vi "Experiment 12.vi"() -> ()   [LabVIEW 2026]
doc: "Experiment 12"
uses:
  <vilib>/AdvancedString/1D String Array to Delimited String (string).vi
  <vilib>/Analysis/baseanly.llb/Mean (DBL).vi
  <vilib>/Analysis/NI_AALBase.lvlib
panel:
  out "No. Of Iterations As Block Of Text (easy to copy into Excel)":string
  out "No. Of Iterations Executed - Loop 10":i32
  out "Output - Loop 10":dbl[](array[numeric]) format="%.3f"
  out "No. Of Iterations Executed - Loop 9":i32
  out "Output - Loop 9":dbl[](array[numeric]) format="%.3f"
  out "No. Of Iterations Executed - Loop 8":i32
  out "Output - Loop 8":dbl[](array[numeric]) format="%.3f"
  out "No. Of Iterations Executed - Loop 7":i32
  out "Output - Loop 7":dbl[](array[numeric]) format="%.3f"
  out "No. Of Iterations Executed - Loop 6":i32
  out "Output - Loop 6":dbl[](array[numeric]) format="%.3f"
  out "No. Of Iterations Executed - Loop 5":i32
  out "Output - Loop 5":dbl[](array[numeric]) format="%.3f"
  out "No. Of Iterations Executed - Loop 4":i32
  out "Output - Loop 4":dbl[](array[numeric]) format="%.3f"
  out "No. Of Iterations Executed - Loop 3":i32
  out "Output - Loop 3":dbl[](array[numeric]) format="%.3f"
  out "Avg. No. Of Iterations Executed - All Loops":dbl format="%.1f"
  out "No. Of Iterations Executed - Loop 2":i32
  out "Output - Loop 2":dbl[](array[numeric]) format="%.3f"
  out "No. Of Iterations Executed - Loop 1":i32
  out "Output - Loop 1":dbl[](array[numeric]) format="%.3f"
  out "Stop VI?":bool
  # "Experiment 12"
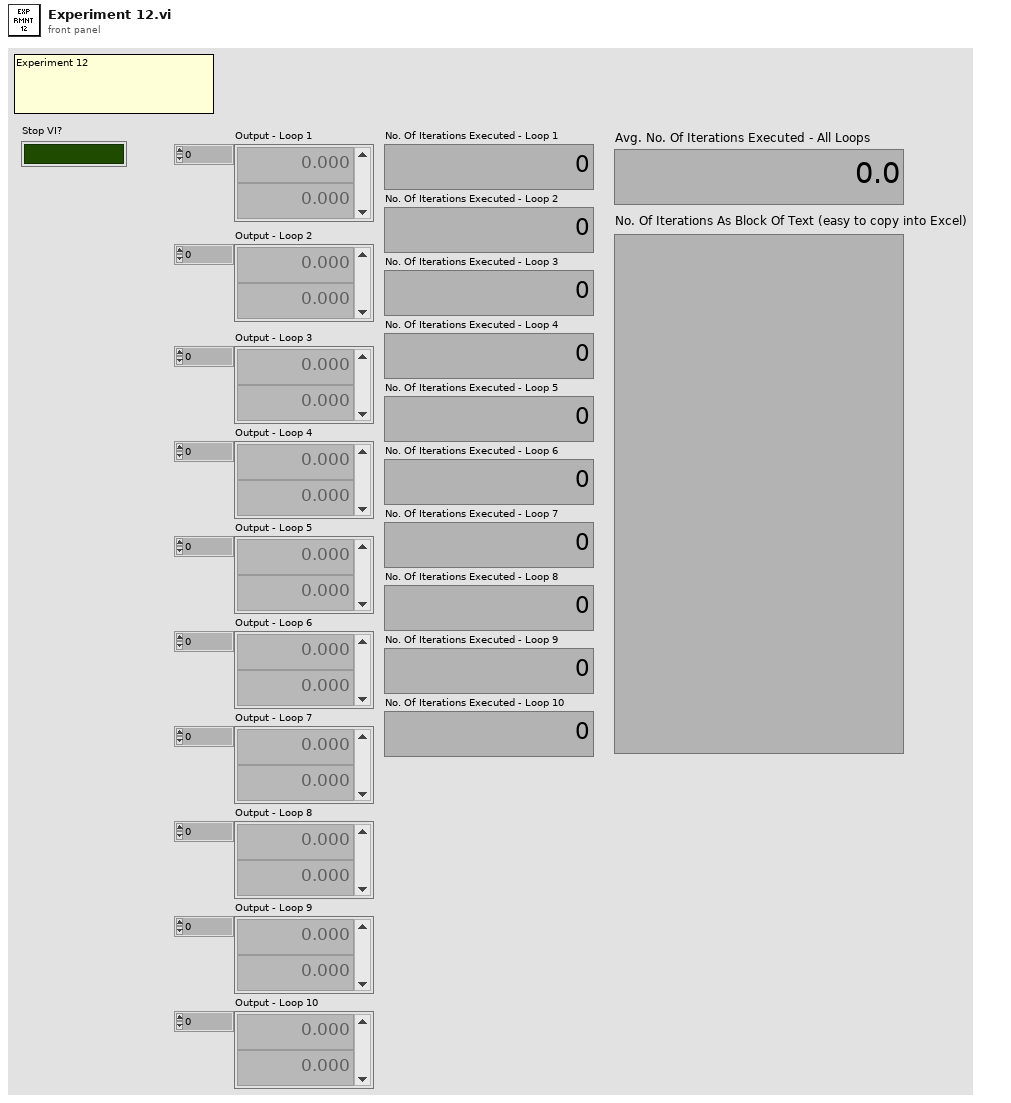
[diagram p1: front panel]
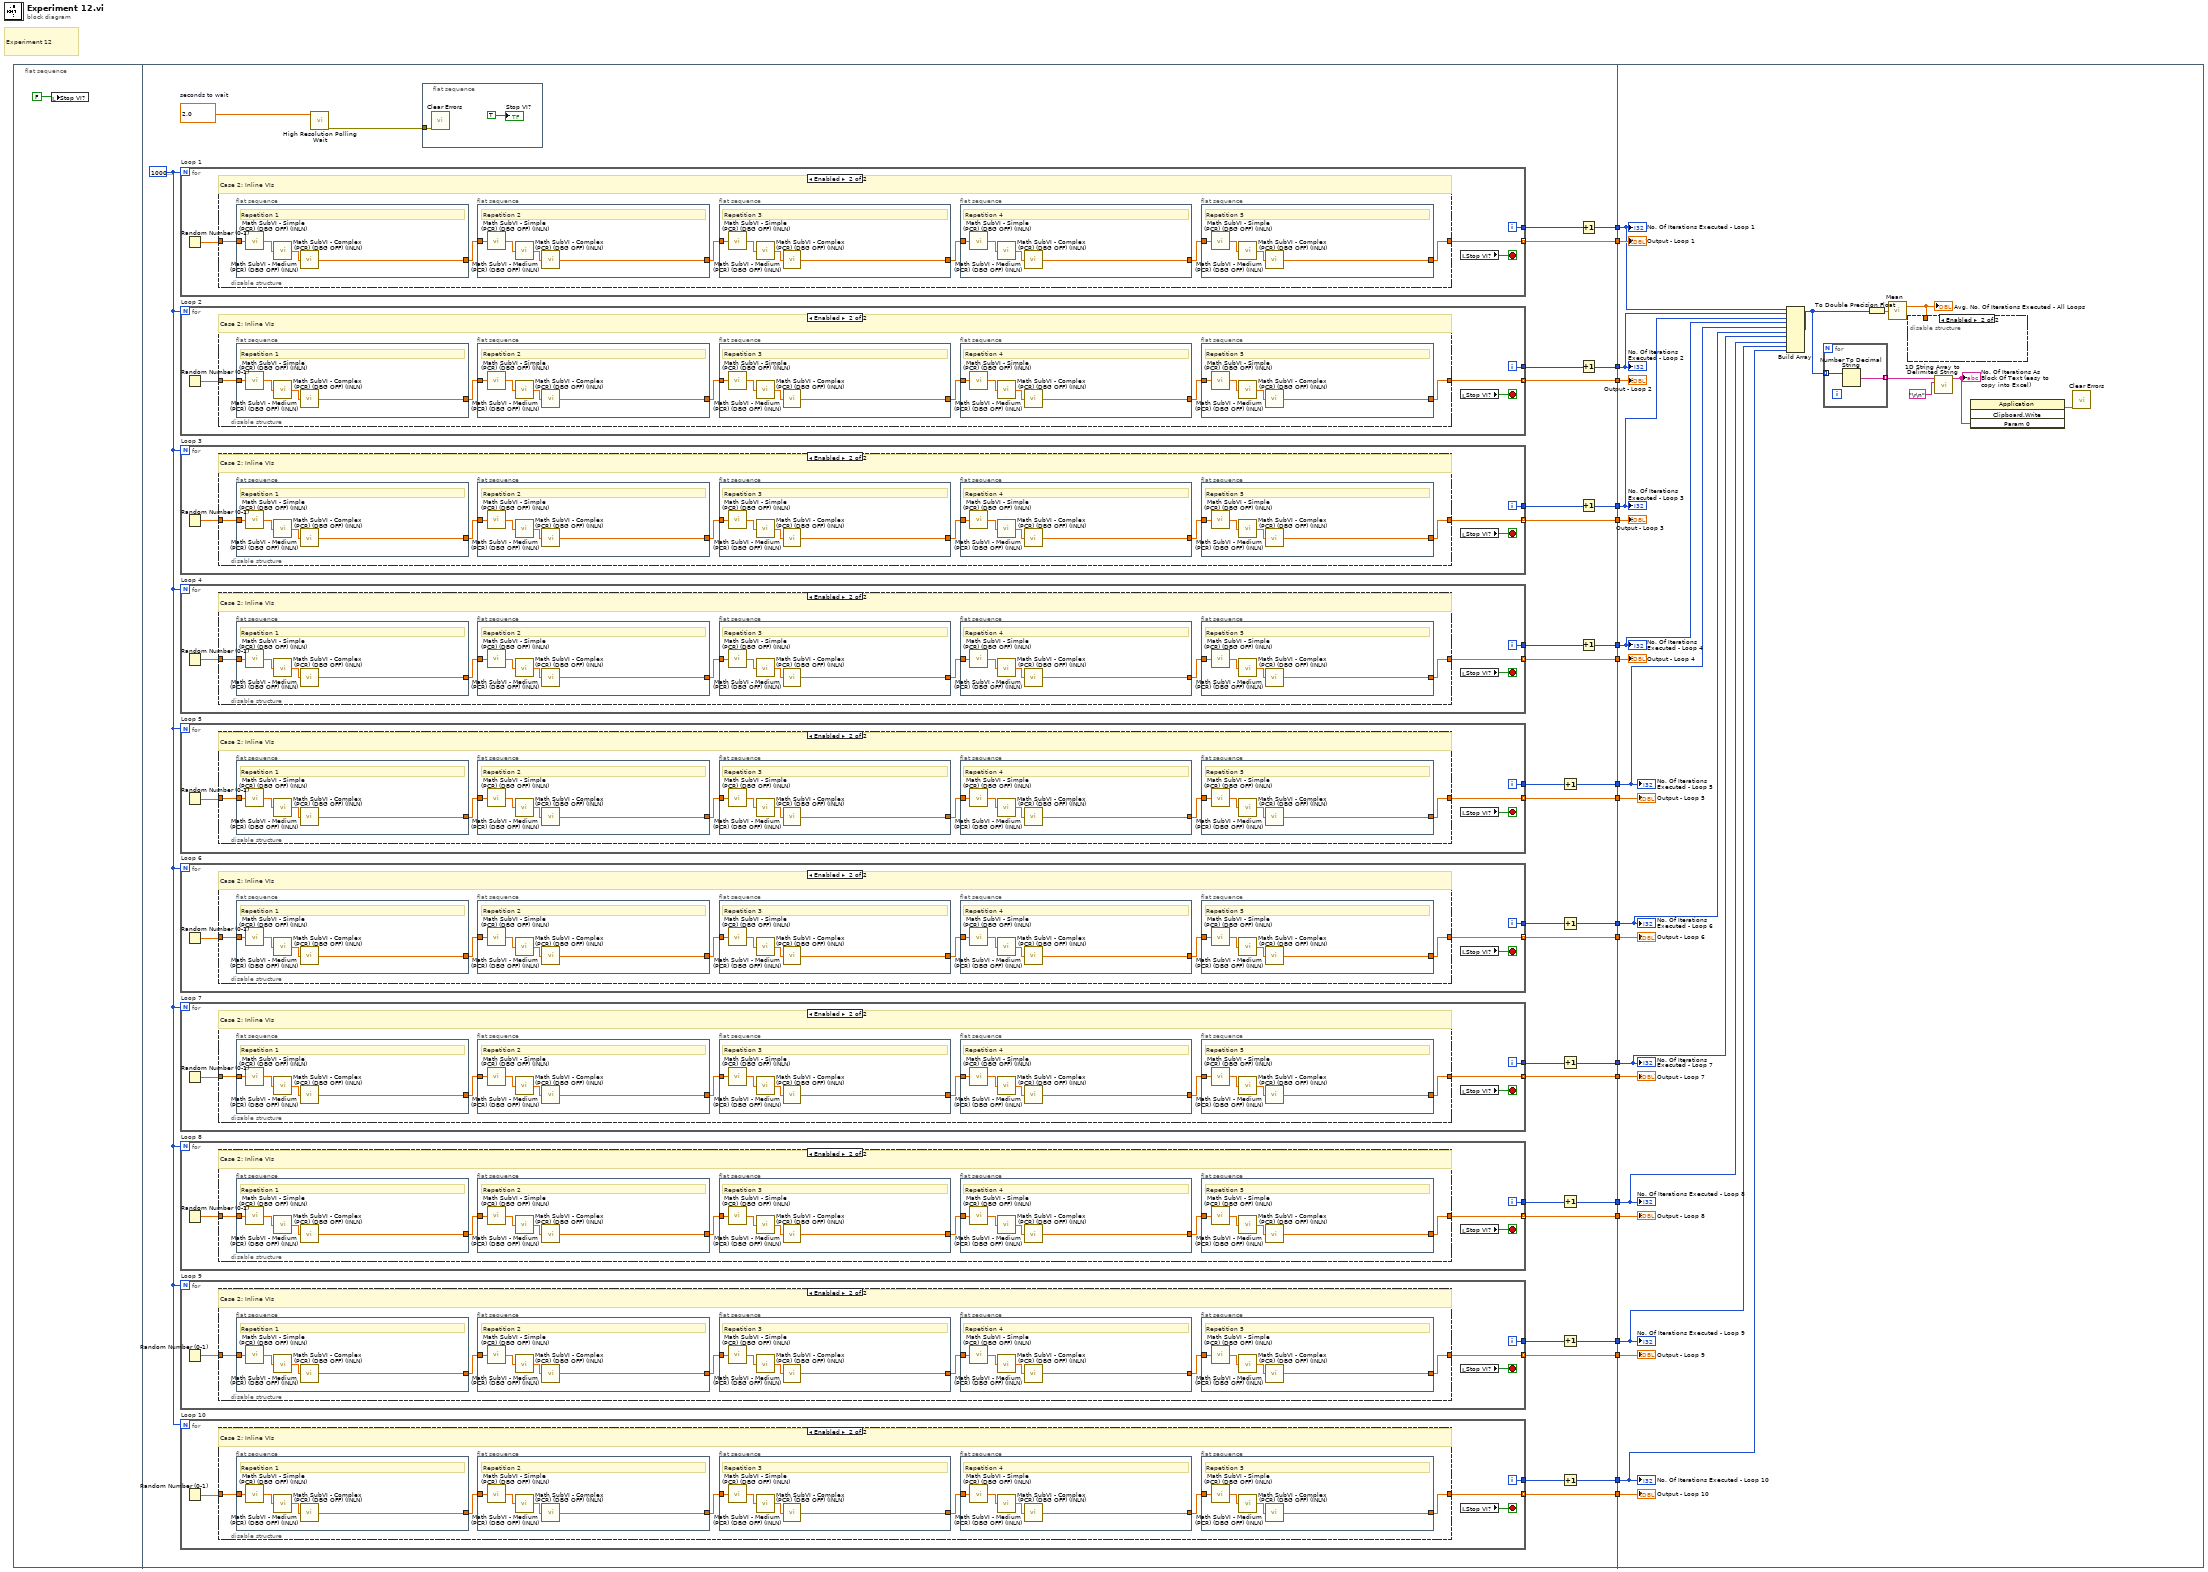
[diagram p0: block diagram]
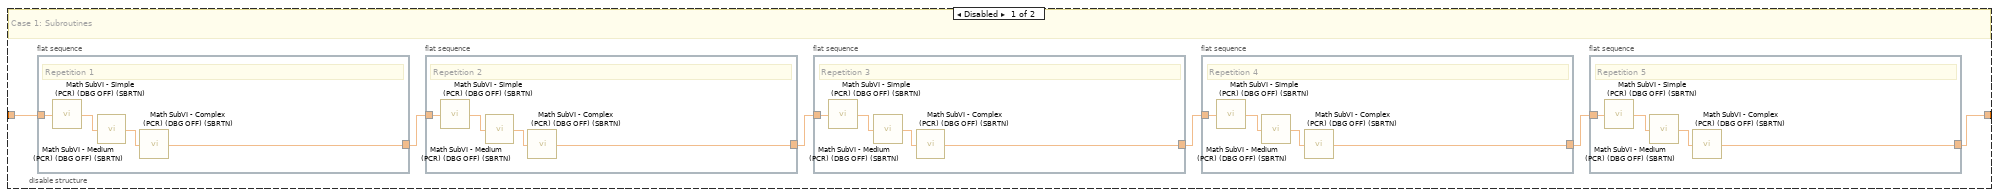
[diagram p2: hidden frame]
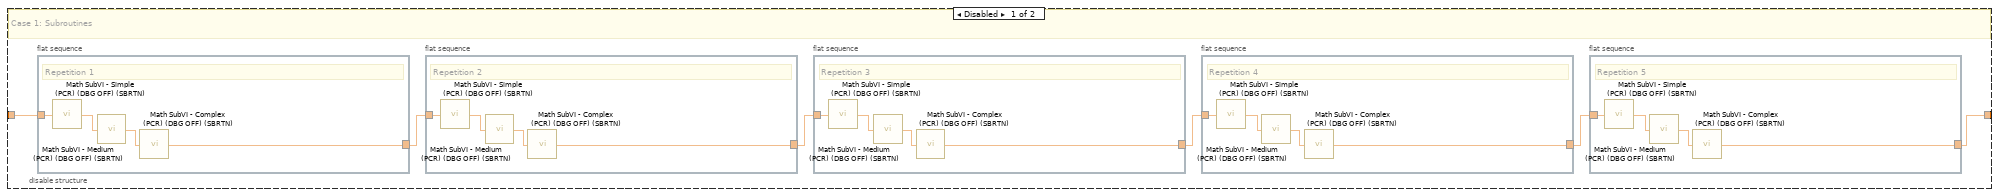
[diagram p3: hidden frame]
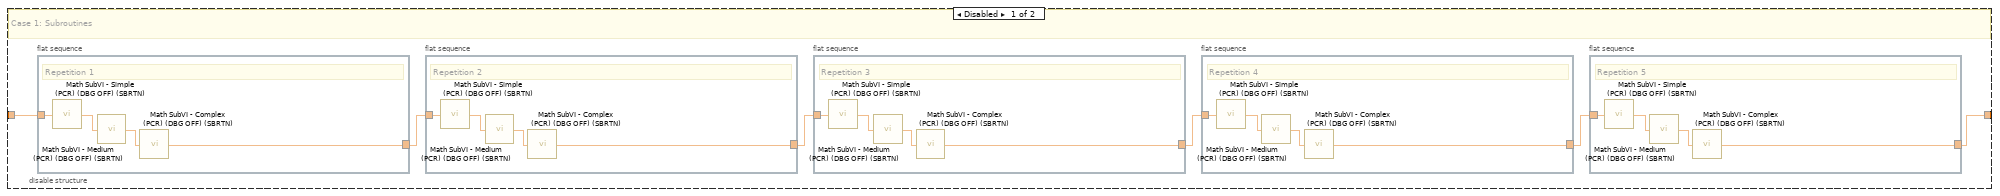
[diagram p4: hidden frame]
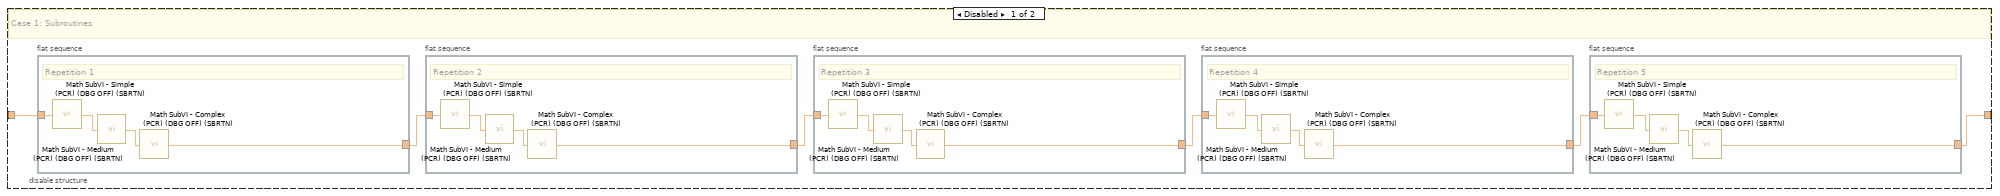
[diagram p5: hidden frame]
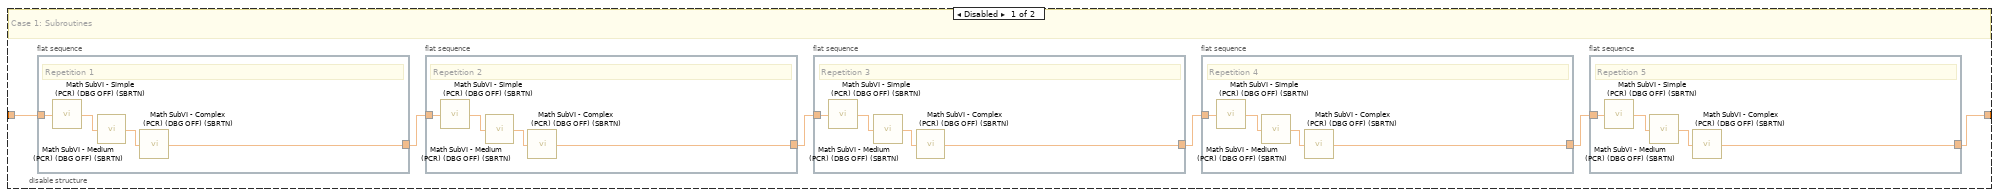
[diagram p6: hidden frame]
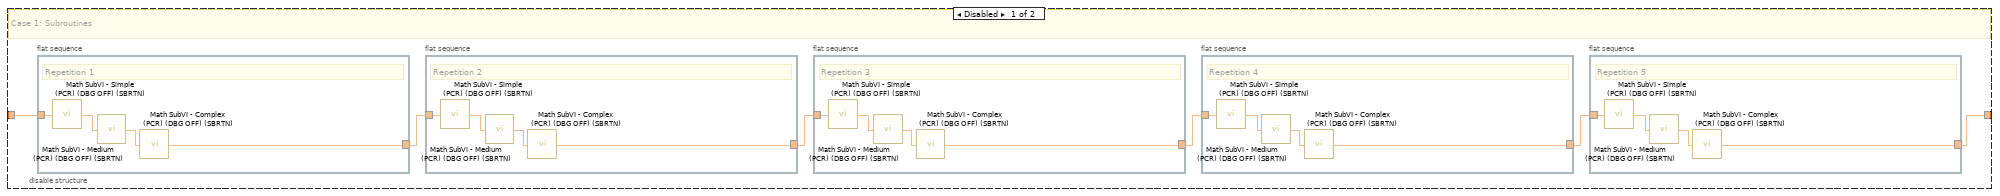
[diagram p7: hidden frame]
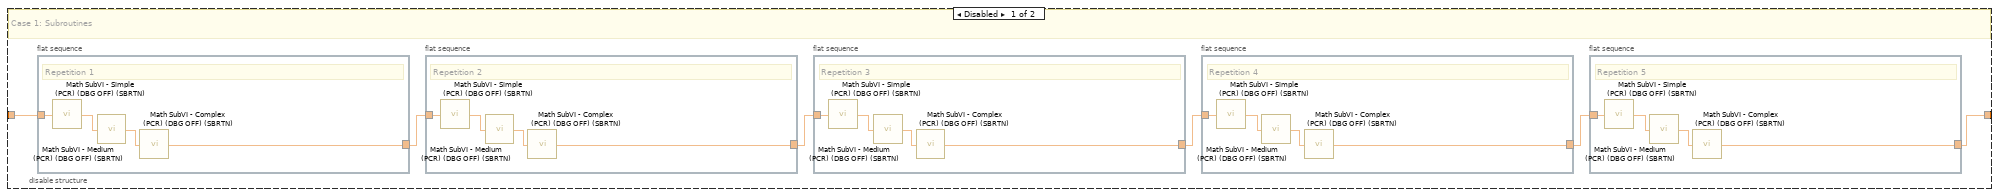
[diagram p8: hidden frame]
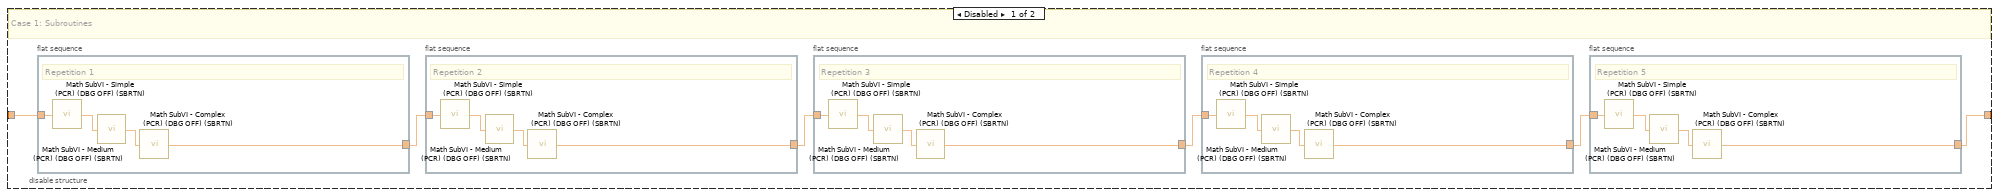
[diagram p9: hidden frame]
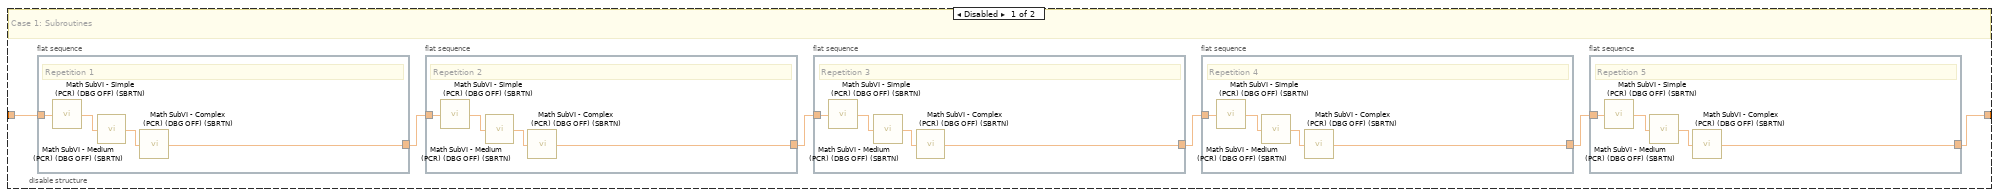
[diagram p10: hidden frame]
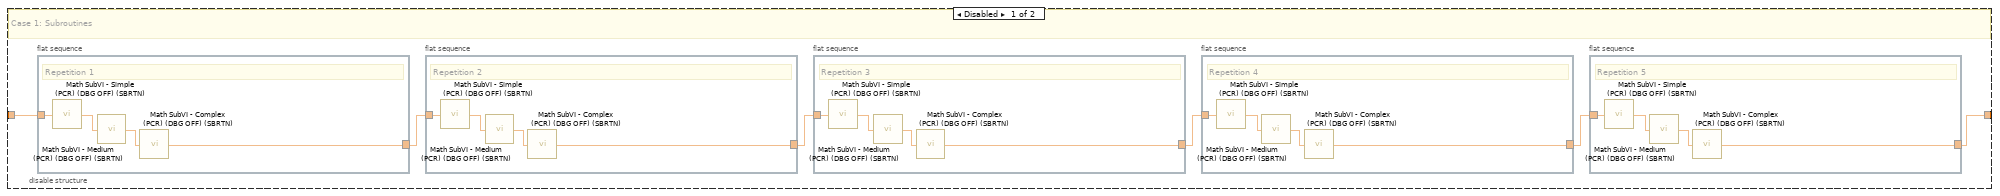
[diagram p11: hidden frame]
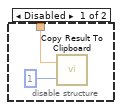
[diagram p12: hidden frame]
diagram:
  # "Experiment 12"
  n1 = flat-sequence {
    tunnel: [w52] -> w20
    tunnel: [w50] -> w19
    tunnel: [w49] -> w18
    tunnel: [w40] -> w17
    tunnel: [w48] -> w16
    tunnel: [w38] -> w15
    tunnel: [w36] -> w14
    tunnel: [w47] -> w13
    tunnel: [w34] -> w12
    tunnel: [w46] -> w11
    tunnel: [w32] -> w10
    tunnel: [w41] -> w9
    tunnel: [w30] -> w8
    tunnel: [w42] -> w7
    tunnel: [w27] -> w6
    tunnel: [w43] -> w5
    tunnel: [w25] -> w4
    tunnel: [w44] -> w3
    tunnel: [w23] -> w2
    tunnel: [w45] -> w1
    tunnel: w20 -> [w643]
    tunnel: w19 -> [w641]
    tunnel: w18 -> [w640]
    tunnel: w17 -> [w642]
    tunnel: w16 -> [w636]
    tunnel: w15 -> [w638]
    tunnel: w14 -> [w637]
    tunnel: w13 -> [w635]
    tunnel: w12 -> [w633]
    tunnel: w11 -> [w627]
    tunnel: w10 -> [w632]
    tunnel: w9 -> [w626]
    tunnel: w8 -> [w631]
    tunnel: w7 -> [w625]
    tunnel: w6 -> [w630]
    tunnel: w5 -> [w624]
    tunnel: w4 -> [w629]
    tunnel: w3 -> [w623]
    tunnel: w2 -> [w628]
    tunnel: w1 -> [w622]
    frame #0 {
      n2 = local write "Stop VI?"(FALSE) -> ()
    }
    frame #1 {
      w22 = 10000000
      w54 = 2.0  # seconds to wait
      n3 = for "Loop 1" {
        N: w22 -> [_]
        tunnel: [w562] -> w52 mode=indexing
        tunnel: [w563] -> w51
        i -> [w563]
        stop <- w564 stop-if-true
        n4 = Random Number (0-1)() -> (number: 0 to 1=w561:dbl)
        n5 = disable-structure shown="Enabled" {
          disable-tunnel: w561 -> [w570 w596]
          disable-tunnel: [w569 w591] -> w562
          frame Disabled {
            # "Case 1: Subroutines"
            n6 = flat-sequence {
              tunnel: w570 -> [w590]
              tunnel: [w587] -> w565
              frame #0 {
                # "Repetition 1"
                n7 = call "Math SubVI - Simple (PCR) (DBG OFF) (SBRTN).vi"("Input"=w590) -> ("Output"=w588:dbl)
                n8 = call "Math SubVI - Medium (PCR) (DBG OFF) (SBRTN).vi"("Input"=w588) -> ("Output"=w589:dbl)
                n9 = call "Math SubVI - Complex (PCR) (DBG OFF) (SBRTN).vi"("Input"=w589) -> ("Output"=w587:dbl)
              }
            }
            n10 = flat-sequence {
              tunnel: w565 -> [w586]
              tunnel: [w583] -> w568
              frame #0 {
                # "Repetition 2"
                n11 = call "Math SubVI - Simple (PCR) (DBG OFF) (SBRTN).vi"("Input"=w586) -> ("Output"=w584:dbl)
                n12 = call "Math SubVI - Medium (PCR) (DBG OFF) (SBRTN).vi"("Input"=w584) -> ("Output"=w585:dbl)
                n13 = call "Math SubVI - Complex (PCR) (DBG OFF) (SBRTN).vi"("Input"=w585) -> ("Output"=w583:dbl)
              }
            }
            n14 = flat-sequence {
              tunnel: w568 -> [w582]
              tunnel: [w579] -> w567
              frame #0 {
                # "Repetition 3"
                n15 = call "Math SubVI - Simple (PCR) (DBG OFF) (SBRTN).vi"("Input"=w582) -> ("Output"=w580:dbl)
                n16 = call "Math SubVI - Medium (PCR) (DBG OFF) (SBRTN).vi"("Input"=w580) -> ("Output"=w581:dbl)
                n17 = call "Math SubVI - Complex (PCR) (DBG OFF) (SBRTN).vi"("Input"=w581) -> ("Output"=w579:dbl)
              }
            }
            n18 = flat-sequence {
              tunnel: w567 -> [w578]
              tunnel: [w575] -> w566
              frame #0 {
                # "Repetition 4"
                n19 = call "Math SubVI - Simple (PCR) (DBG OFF) (SBRTN).vi"("Input"=w578) -> ("Output"=w576:dbl)
                n20 = call "Math SubVI - Medium (PCR) (DBG OFF) (SBRTN).vi"("Input"=w576) -> ("Output"=w577:dbl)
                n21 = call "Math SubVI - Complex (PCR) (DBG OFF) (SBRTN).vi"("Input"=w577) -> ("Output"=w575:dbl)
              }
            }
            n22 = flat-sequence {
              tunnel: w566 -> [w574]
              tunnel: [w571] -> w569
              frame #0 {
                # "Repetition 5"
                n23 = call "Math SubVI - Simple (PCR) (DBG OFF) (SBRTN).vi"("Input"=w574) -> ("Output"=w572:dbl)
                n24 = call "Math SubVI - Medium (PCR) (DBG OFF) (SBRTN).vi"("Input"=w572) -> ("Output"=w573:dbl)
                n25 = call "Math SubVI - Complex (PCR) (DBG OFF) (SBRTN).vi"("Input"=w573) -> ("Output"=w571:dbl)
              }
            }
          }
          frame Enabled {
            # "Case 2: Inline VIs"
            n26 = flat-sequence {
              tunnel: w596 -> [w616]
              tunnel: [w613] -> w595
              frame #0 {
                # "Repetition 1"
                n27 = call "Math SubVI - Simple (PCR) (DBG OFF) (INLN).vi"("Input"=w616) -> ("Output"=w614:dbl)
                n28 = call "Math SubVI - Medium (PCR) (DBG OFF) (INLN).vi"("Input"=w614) -> ("Output"=w615:dbl)
                n29 = call "Math SubVI - Complex (PCR) (DBG OFF) (INLN).vi"("Input"=w615) -> ("Output"=w613:dbl)
              }
            }
            n30 = flat-sequence {
              tunnel: w595 -> [w612]
              tunnel: [w609] -> w594
              frame #0 {
                # "Repetition 2"
                n31 = call "Math SubVI - Simple (PCR) (DBG OFF) (INLN).vi"("Input"=w612) -> ("Output"=w610:dbl)
                n32 = call "Math SubVI - Medium (PCR) (DBG OFF) (INLN).vi"("Input"=w610) -> ("Output"=w611:dbl)
                n33 = call "Math SubVI - Complex (PCR) (DBG OFF) (INLN).vi"("Input"=w611) -> ("Output"=w609:dbl)
              }
            }
            n34 = flat-sequence {
              tunnel: w594 -> [w608]
              tunnel: [w605] -> w593
              frame #0 {
                # "Repetition 3"
                n35 = call "Math SubVI - Simple (PCR) (DBG OFF) (INLN).vi"("Input"=w608) -> ("Output"=w606:dbl)
                n36 = call "Math SubVI - Medium (PCR) (DBG OFF) (INLN).vi"("Input"=w606) -> ("Output"=w607:dbl)
                n37 = call "Math SubVI - Complex (PCR) (DBG OFF) (INLN).vi"("Input"=w607) -> ("Output"=w605:dbl)
              }
            }
            n38 = flat-sequence {
              tunnel: w593 -> [w604]
              tunnel: [w601] -> w592
              frame #0 {
                # "Repetition 4"
                n39 = call "Math SubVI - Simple (PCR) (DBG OFF) (INLN).vi"("Input"=w604) -> ("Output"=w602:dbl)
                n40 = call "Math SubVI - Medium (PCR) (DBG OFF) (INLN).vi"("Input"=w602) -> ("Output"=w603:dbl)
                n41 = call "Math SubVI - Complex (PCR) (DBG OFF) (INLN).vi"("Input"=w603) -> ("Output"=w601:dbl)
              }
            }
            n42 = flat-sequence {
              tunnel: w592 -> [w600]
              tunnel: [w597] -> w591
              frame #0 {
                # "Repetition 5"
                n43 = call "Math SubVI - Simple (PCR) (DBG OFF) (INLN).vi"("Input"=w600) -> ("Output"=w598:dbl)
                n44 = call "Math SubVI - Medium (PCR) (DBG OFF) (INLN).vi"("Input"=w598) -> ("Output"=w599:dbl)
                n45 = call "Math SubVI - Complex (PCR) (DBG OFF) (INLN).vi"("Input"=w599) -> ("Output"=w597:dbl)
              }
            }
          }
        }
        n46 = local read "Stop VI?"() -> (w564:bool)
      }
      n47 = for "Loop 2" {
        N: w22 -> [_]
        tunnel: [w506] -> w40 mode=indexing
        tunnel: [w507] -> w39
        i -> [w507]
        stop <- w508 stop-if-true
        n48 = Random Number (0-1)() -> (number: 0 to 1=w505:dbl)
        n49 = disable-structure shown="Enabled" {
          disable-tunnel: w505 -> [w514 w540]
          disable-tunnel: [w513 w535] -> w506
          frame Disabled {
            # "Case 1: Subroutines"
            n50 = flat-sequence {
              tunnel: w514 -> [w534]
              tunnel: [w531] -> w509
              frame #0 {
                # "Repetition 1"
                n51 = call "Math SubVI - Simple (PCR) (DBG OFF) (SBRTN).vi"("Input"=w534) -> ("Output"=w532:dbl)
                n52 = call "Math SubVI - Medium (PCR) (DBG OFF) (SBRTN).vi"("Input"=w532) -> ("Output"=w533:dbl)
                n53 = call "Math SubVI - Complex (PCR) (DBG OFF) (SBRTN).vi"("Input"=w533) -> ("Output"=w531:dbl)
              }
            }
            n54 = flat-sequence {
              tunnel: w509 -> [w530]
              tunnel: [w527] -> w512
              frame #0 {
                # "Repetition 2"
                n55 = call "Math SubVI - Simple (PCR) (DBG OFF) (SBRTN).vi"("Input"=w530) -> ("Output"=w528:dbl)
                n56 = call "Math SubVI - Medium (PCR) (DBG OFF) (SBRTN).vi"("Input"=w528) -> ("Output"=w529:dbl)
                n57 = call "Math SubVI - Complex (PCR) (DBG OFF) (SBRTN).vi"("Input"=w529) -> ("Output"=w527:dbl)
              }
            }
            n58 = flat-sequence {
              tunnel: w512 -> [w526]
              tunnel: [w523] -> w511
              frame #0 {
                # "Repetition 3"
                n59 = call "Math SubVI - Simple (PCR) (DBG OFF) (SBRTN).vi"("Input"=w526) -> ("Output"=w524:dbl)
                n60 = call "Math SubVI - Medium (PCR) (DBG OFF) (SBRTN).vi"("Input"=w524) -> ("Output"=w525:dbl)
                n61 = call "Math SubVI - Complex (PCR) (DBG OFF) (SBRTN).vi"("Input"=w525) -> ("Output"=w523:dbl)
              }
            }
            n62 = flat-sequence {
              tunnel: w511 -> [w522]
              tunnel: [w519] -> w510
              frame #0 {
                # "Repetition 4"
                n63 = call "Math SubVI - Simple (PCR) (DBG OFF) (SBRTN).vi"("Input"=w522) -> ("Output"=w520:dbl)
                n64 = call "Math SubVI - Medium (PCR) (DBG OFF) (SBRTN).vi"("Input"=w520) -> ("Output"=w521:dbl)
                n65 = call "Math SubVI - Complex (PCR) (DBG OFF) (SBRTN).vi"("Input"=w521) -> ("Output"=w519:dbl)
              }
            }
            n66 = flat-sequence {
              tunnel: w510 -> [w518]
              tunnel: [w515] -> w513
              frame #0 {
                # "Repetition 5"
                n67 = call "Math SubVI - Simple (PCR) (DBG OFF) (SBRTN).vi"("Input"=w518) -> ("Output"=w516:dbl)
                n68 = call "Math SubVI - Medium (PCR) (DBG OFF) (SBRTN).vi"("Input"=w516) -> ("Output"=w517:dbl)
                n69 = call "Math SubVI - Complex (PCR) (DBG OFF) (SBRTN).vi"("Input"=w517) -> ("Output"=w515:dbl)
              }
            }
          }
          frame Enabled {
            # "Case 2: Inline VIs"
            n70 = flat-sequence {
              tunnel: w540 -> [w560]
              tunnel: [w557] -> w539
              frame #0 {
                # "Repetition 1"
                n71 = call "Math SubVI - Simple (PCR) (DBG OFF) (INLN).vi"("Input"=w560) -> ("Output"=w558:dbl)
                n72 = call "Math SubVI - Medium (PCR) (DBG OFF) (INLN).vi"("Input"=w558) -> ("Output"=w559:dbl)
                n73 = call "Math SubVI - Complex (PCR) (DBG OFF) (INLN).vi"("Input"=w559) -> ("Output"=w557:dbl)
              }
            }
            n74 = flat-sequence {
              tunnel: w539 -> [w556]
              tunnel: [w553] -> w538
              frame #0 {
                # "Repetition 2"
                n75 = call "Math SubVI - Simple (PCR) (DBG OFF) (INLN).vi"("Input"=w556) -> ("Output"=w554:dbl)
                n76 = call "Math SubVI - Medium (PCR) (DBG OFF) (INLN).vi"("Input"=w554) -> ("Output"=w555:dbl)
                n77 = call "Math SubVI - Complex (PCR) (DBG OFF) (INLN).vi"("Input"=w555) -> ("Output"=w553:dbl)
              }
            }
            n78 = flat-sequence {
              tunnel: w538 -> [w552]
              tunnel: [w549] -> w537
              frame #0 {
                # "Repetition 3"
                n79 = call "Math SubVI - Simple (PCR) (DBG OFF) (INLN).vi"("Input"=w552) -> ("Output"=w550:dbl)
                n80 = call "Math SubVI - Medium (PCR) (DBG OFF) (INLN).vi"("Input"=w550) -> ("Output"=w551:dbl)
                n81 = call "Math SubVI - Complex (PCR) (DBG OFF) (INLN).vi"("Input"=w551) -> ("Output"=w549:dbl)
              }
            }
            n82 = flat-sequence {
              tunnel: w537 -> [w548]
              tunnel: [w545] -> w536
              frame #0 {
                # "Repetition 4"
                n83 = call "Math SubVI - Simple (PCR) (DBG OFF) (INLN).vi"("Input"=w548) -> ("Output"=w546:dbl)
                n84 = call "Math SubVI - Medium (PCR) (DBG OFF) (INLN).vi"("Input"=w546) -> ("Output"=w547:dbl)
                n85 = call "Math SubVI - Complex (PCR) (DBG OFF) (INLN).vi"("Input"=w547) -> ("Output"=w545:dbl)
              }
            }
            n86 = flat-sequence {
              tunnel: w536 -> [w544]
              tunnel: [w541] -> w535
              frame #0 {
                # "Repetition 5"
                n87 = call "Math SubVI - Simple (PCR) (DBG OFF) (INLN).vi"("Input"=w544) -> ("Output"=w542:dbl)
                n88 = call "Math SubVI - Medium (PCR) (DBG OFF) (INLN).vi"("Input"=w542) -> ("Output"=w543:dbl)
                n89 = call "Math SubVI - Complex (PCR) (DBG OFF) (INLN).vi"("Input"=w543) -> ("Output"=w541:dbl)
              }
            }
          }
        }
        n90 = local read "Stop VI?"() -> (w508:bool)
      }
      n91 = for "Loop 3" {
        N: w22 -> [_]
        tunnel: [w450] -> w38 mode=indexing
        tunnel: [w451] -> w37
        i -> [w451]
        stop <- w452 stop-if-true
        n92 = Random Number (0-1)() -> (number: 0 to 1=w449:dbl)
        n93 = disable-structure shown="Enabled" {
          disable-tunnel: w449 -> [w458 w484]
          disable-tunnel: [w457 w479] -> w450
          frame Disabled {
            # "Case 1: Subroutines"
            n94 = flat-sequence {
              tunnel: w458 -> [w478]
              tunnel: [w475] -> w453
              frame #0 {
                # "Repetition 1"
                n95 = call "Math SubVI - Simple (PCR) (DBG OFF) (SBRTN).vi"("Input"=w478) -> ("Output"=w476:dbl)
                n96 = call "Math SubVI - Medium (PCR) (DBG OFF) (SBRTN).vi"("Input"=w476) -> ("Output"=w477:dbl)
                n97 = call "Math SubVI - Complex (PCR) (DBG OFF) (SBRTN).vi"("Input"=w477) -> ("Output"=w475:dbl)
              }
            }
            n98 = flat-sequence {
              tunnel: w453 -> [w474]
              tunnel: [w471] -> w456
              frame #0 {
                # "Repetition 2"
                n99 = call "Math SubVI - Simple (PCR) (DBG OFF) (SBRTN).vi"("Input"=w474) -> ("Output"=w472:dbl)
                n100 = call "Math SubVI - Medium (PCR) (DBG OFF) (SBRTN).vi"("Input"=w472) -> ("Output"=w473:dbl)
                n101 = call "Math SubVI - Complex (PCR) (DBG OFF) (SBRTN).vi"("Input"=w473) -> ("Output"=w471:dbl)
              }
            }
            n102 = flat-sequence {
              tunnel: w456 -> [w470]
              tunnel: [w467] -> w455
              frame #0 {
                # "Repetition 3"
                n103 = call "Math SubVI - Simple (PCR) (DBG OFF) (SBRTN).vi"("Input"=w470) -> ("Output"=w468:dbl)
                n104 = call "Math SubVI - Medium (PCR) (DBG OFF) (SBRTN).vi"("Input"=w468) -> ("Output"=w469:dbl)
                n105 = call "Math SubVI - Complex (PCR) (DBG OFF) (SBRTN).vi"("Input"=w469) -> ("Output"=w467:dbl)
              }
            }
            n106 = flat-sequence {
              tunnel: w455 -> [w466]
              tunnel: [w463] -> w454
              frame #0 {
                # "Repetition 4"
                n107 = call "Math SubVI - Simple (PCR) (DBG OFF) (SBRTN).vi"("Input"=w466) -> ("Output"=w464:dbl)
                n108 = call "Math SubVI - Medium (PCR) (DBG OFF) (SBRTN).vi"("Input"=w464) -> ("Output"=w465:dbl)
                n109 = call "Math SubVI - Complex (PCR) (DBG OFF) (SBRTN).vi"("Input"=w465) -> ("Output"=w463:dbl)
              }
            }
            n110 = flat-sequence {
              tunnel: w454 -> [w462]
              tunnel: [w459] -> w457
              frame #0 {
                # "Repetition 5"
                n111 = call "Math SubVI - Simple (PCR) (DBG OFF) (SBRTN).vi"("Input"=w462) -> ("Output"=w460:dbl)
                n112 = call "Math SubVI - Medium (PCR) (DBG OFF) (SBRTN).vi"("Input"=w460) -> ("Output"=w461:dbl)
                n113 = call "Math SubVI - Complex (PCR) (DBG OFF) (SBRTN).vi"("Input"=w461) -> ("Output"=w459:dbl)
              }
            }
          }
          frame Enabled {
            # "Case 2: Inline VIs"
            n114 = flat-sequence {
              tunnel: w484 -> [w504]
              tunnel: [w501] -> w483
              frame #0 {
                # "Repetition 1"
                n115 = call "Math SubVI - Simple (PCR) (DBG OFF) (INLN).vi"("Input"=w504) -> ("Output"=w502:dbl)
                n116 = call "Math SubVI - Medium (PCR) (DBG OFF) (INLN).vi"("Input"=w502) -> ("Output"=w503:dbl)
                n117 = call "Math SubVI - Complex (PCR) (DBG OFF) (INLN).vi"("Input"=w503) -> ("Output"=w501:dbl)
              }
            }
            n118 = flat-sequence {
              tunnel: w483 -> [w500]
              tunnel: [w497] -> w482
              frame #0 {
                # "Repetition 2"
                n119 = call "Math SubVI - Simple (PCR) (DBG OFF) (INLN).vi"("Input"=w500) -> ("Output"=w498:dbl)
                n120 = call "Math SubVI - Medium (PCR) (DBG OFF) (INLN).vi"("Input"=w498) -> ("Output"=w499:dbl)
                n121 = call "Math SubVI - Complex (PCR) (DBG OFF) (INLN).vi"("Input"=w499) -> ("Output"=w497:dbl)
              }
            }
            n122 = flat-sequence {
              tunnel: w482 -> [w496]
              tunnel: [w493] -> w481
              frame #0 {
                # "Repetition 3"
                n123 = call "Math SubVI - Simple (PCR) (DBG OFF) (INLN).vi"("Input"=w496) -> ("Output"=w494:dbl)
                n124 = call "Math SubVI - Medium (PCR) (DBG OFF) (INLN).vi"("Input"=w494) -> ("Output"=w495:dbl)
                n125 = call "Math SubVI - Complex (PCR) (DBG OFF) (INLN).vi"("Input"=w495) -> ("Output"=w493:dbl)
              }
            }
            n126 = flat-sequence {
              tunnel: w481 -> [w492]
              tunnel: [w489] -> w480
              frame #0 {
                # "Repetition 4"
                n127 = call "Math SubVI - Simple (PCR) (DBG OFF) (INLN).vi"("Input"=w492) -> ("Output"=w490:dbl)
                n128 = call "Math SubVI - Medium (PCR) (DBG OFF) (INLN).vi"("Input"=w490) -> ("Output"=w491:dbl)
                n129 = call "Math SubVI - Complex (PCR) (DBG OFF) (INLN).vi"("Input"=w491) -> ("Output"=w489:dbl)
              }
            }
            n130 = flat-sequence {
              tunnel: w480 -> [w488]
              tunnel: [w485] -> w479
              frame #0 {
                # "Repetition 5"
                n131 = call "Math SubVI - Simple (PCR) (DBG OFF) (INLN).vi"("Input"=w488) -> ("Output"=w486:dbl)
                n132 = call "Math SubVI - Medium (PCR) (DBG OFF) (INLN).vi"("Input"=w486) -> ("Output"=w487:dbl)
                n133 = call "Math SubVI - Complex (PCR) (DBG OFF) (INLN).vi"("Input"=w487) -> ("Output"=w485:dbl)
              }
            }
          }
        }
        n134 = local read "Stop VI?"() -> (w452:bool)
      }
      n135 = for "Loop 4" {
        N: w22 -> [_]
        tunnel: [w394] -> w36 mode=indexing
        tunnel: [w395] -> w35
        i -> [w395]
        stop <- w396 stop-if-true
        n136 = Random Number (0-1)() -> (number: 0 to 1=w393:dbl)
        n137 = disable-structure shown="Enabled" {
          disable-tunnel: w393 -> [w402 w428]
          disable-tunnel: [w401 w423] -> w394
          frame Disabled {
            # "Case 1: Subroutines"
            n138 = flat-sequence {
              tunnel: w402 -> [w422]
              tunnel: [w419] -> w397
              frame #0 {
                # "Repetition 1"
                n139 = call "Math SubVI - Simple (PCR) (DBG OFF) (SBRTN).vi"("Input"=w422) -> ("Output"=w420:dbl)
                n140 = call "Math SubVI - Medium (PCR) (DBG OFF) (SBRTN).vi"("Input"=w420) -> ("Output"=w421:dbl)
                n141 = call "Math SubVI - Complex (PCR) (DBG OFF) (SBRTN).vi"("Input"=w421) -> ("Output"=w419:dbl)
              }
            }
            n142 = flat-sequence {
              tunnel: w397 -> [w418]
              tunnel: [w415] -> w400
              frame #0 {
                # "Repetition 2"
                n143 = call "Math SubVI - Simple (PCR) (DBG OFF) (SBRTN).vi"("Input"=w418) -> ("Output"=w416:dbl)
                n144 = call "Math SubVI - Medium (PCR) (DBG OFF) (SBRTN).vi"("Input"=w416) -> ("Output"=w417:dbl)
                n145 = call "Math SubVI - Complex (PCR) (DBG OFF) (SBRTN).vi"("Input"=w417) -> ("Output"=w415:dbl)
              }
            }
            n146 = flat-sequence {
              tunnel: w400 -> [w414]
              tunnel: [w411] -> w399
              frame #0 {
                # "Repetition 3"
                n147 = call "Math SubVI - Simple (PCR) (DBG OFF) (SBRTN).vi"("Input"=w414) -> ("Output"=w412:dbl)
                n148 = call "Math SubVI - Medium (PCR) (DBG OFF) (SBRTN).vi"("Input"=w412) -> ("Output"=w413:dbl)
                n149 = call "Math SubVI - Complex (PCR) (DBG OFF) (SBRTN).vi"("Input"=w413) -> ("Output"=w411:dbl)
              }
            }
            n150 = flat-sequence {
              tunnel: w399 -> [w410]
              tunnel: [w407] -> w398
              frame #0 {
                # "Repetition 4"
                n151 = call "Math SubVI - Simple (PCR) (DBG OFF) (SBRTN).vi"("Input"=w410) -> ("Output"=w408:dbl)
                n152 = call "Math SubVI - Medium (PCR) (DBG OFF) (SBRTN).vi"("Input"=w408) -> ("Output"=w409:dbl)
                n153 = call "Math SubVI - Complex (PCR) (DBG OFF) (SBRTN).vi"("Input"=w409) -> ("Output"=w407:dbl)
              }
            }
            n154 = flat-sequence {
              tunnel: w398 -> [w406]
              tunnel: [w403] -> w401
              frame #0 {
                # "Repetition 5"
                n155 = call "Math SubVI - Simple (PCR) (DBG OFF) (SBRTN).vi"("Input"=w406) -> ("Output"=w404:dbl)
                n156 = call "Math SubVI - Medium (PCR) (DBG OFF) (SBRTN).vi"("Input"=w404) -> ("Output"=w405:dbl)
                n157 = call "Math SubVI - Complex (PCR) (DBG OFF) (SBRTN).vi"("Input"=w405) -> ("Output"=w403:dbl)
              }
            }
          }
          frame Enabled {
            # "Case 2: Inline VIs"
            n158 = flat-sequence {
              tunnel: w428 -> [w448]
              tunnel: [w445] -> w427
              frame #0 {
                # "Repetition 1"
                n159 = call "Math SubVI - Simple (PCR) (DBG OFF) (INLN).vi"("Input"=w448) -> ("Output"=w446:dbl)
                n160 = call "Math SubVI - Medium (PCR) (DBG OFF) (INLN).vi"("Input"=w446) -> ("Output"=w447:dbl)
                n161 = call "Math SubVI - Complex (PCR) (DBG OFF) (INLN).vi"("Input"=w447) -> ("Output"=w445:dbl)
              }
            }
            n162 = flat-sequence {
              tunnel: w427 -> [w444]
              tunnel: [w441] -> w426
              frame #0 {
                # "Repetition 2"
                n163 = call "Math SubVI - Simple (PCR) (DBG OFF) (INLN).vi"("Input"=w444) -> ("Output"=w442:dbl)
                n164 = call "Math SubVI - Medium (PCR) (DBG OFF) (INLN).vi"("Input"=w442) -> ("Output"=w443:dbl)
                n165 = call "Math SubVI - Complex (PCR) (DBG OFF) (INLN).vi"("Input"=w443) -> ("Output"=w441:dbl)
              }
            }
            n166 = flat-sequence {
              tunnel: w426 -> [w440]
              tunnel: [w437] -> w425
              frame #0 {
                # "Repetition 3"
                n167 = call "Math SubVI - Simple (PCR) (DBG OFF) (INLN).vi"("Input"=w440) -> ("Output"=w438:dbl)
                n168 = call "Math SubVI - Medium (PCR) (DBG OFF) (INLN).vi"("Input"=w438) -> ("Output"=w439:dbl)
                n169 = call "Math SubVI - Complex (PCR) (DBG OFF) (INLN).vi"("Input"=w439) -> ("Output"=w437:dbl)
              }
            }
            n170 = flat-sequence {
              tunnel: w425 -> [w436]
              tunnel: [w433] -> w424
              frame #0 {
                # "Repetition 4"
                n171 = call "Math SubVI - Simple (PCR) (DBG OFF) (INLN).vi"("Input"=w436) -> ("Output"=w434:dbl)
                n172 = call "Math SubVI - Medium (PCR) (DBG OFF) (INLN).vi"("Input"=w434) -> ("Output"=w435:dbl)
                n173 = call "Math SubVI - Complex (PCR) (DBG OFF) (INLN).vi"("Input"=w435) -> ("Output"=w433:dbl)
              }
            }
            n174 = flat-sequence {
              tunnel: w424 -> [w432]
              tunnel: [w429] -> w423
              frame #0 {
                # "Repetition 5"
                n175 = call "Math SubVI - Simple (PCR) (DBG OFF) (INLN).vi"("Input"=w432) -> ("Output"=w430:dbl)
                n176 = call "Math SubVI - Medium (PCR) (DBG OFF) (INLN).vi"("Input"=w430) -> ("Output"=w431:dbl)
                n177 = call "Math SubVI - Complex (PCR) (DBG OFF) (INLN).vi"("Input"=w431) -> ("Output"=w429:dbl)
              }
            }
          }
        }
        n178 = local read "Stop VI?"() -> (w396:bool)
      }
      n179 = for "Loop 5" {
        N: w22 -> [_]
        tunnel: [w338] -> w34 mode=indexing
        tunnel: [w339] -> w33
        i -> [w339]
        stop <- w340 stop-if-true
        n180 = Random Number (0-1)() -> (number: 0 to 1=w337:dbl)
        n181 = disable-structure shown="Enabled" {
          disable-tunnel: w337 -> [w346 w372]
          disable-tunnel: [w345 w367] -> w338
          frame Disabled {
            # "Case 1: Subroutines"
            n182 = flat-sequence {
              tunnel: w346 -> [w366]
              tunnel: [w363] -> w341
              frame #0 {
                # "Repetition 1"
                n183 = call "Math SubVI - Simple (PCR) (DBG OFF) (SBRTN).vi"("Input"=w366) -> ("Output"=w364:dbl)
                n184 = call "Math SubVI - Medium (PCR) (DBG OFF) (SBRTN).vi"("Input"=w364) -> ("Output"=w365:dbl)
                n185 = call "Math SubVI - Complex (PCR) (DBG OFF) (SBRTN).vi"("Input"=w365) -> ("Output"=w363:dbl)
              }
            }
            n186 = flat-sequence {
              tunnel: w341 -> [w362]
              tunnel: [w359] -> w344
              frame #0 {
                # "Repetition 2"
                n187 = call "Math SubVI - Simple (PCR) (DBG OFF) (SBRTN).vi"("Input"=w362) -> ("Output"=w360:dbl)
                n188 = call "Math SubVI - Medium (PCR) (DBG OFF) (SBRTN).vi"("Input"=w360) -> ("Output"=w361:dbl)
                n189 = call "Math SubVI - Complex (PCR) (DBG OFF) (SBRTN).vi"("Input"=w361) -> ("Output"=w359:dbl)
              }
            }
            n190 = flat-sequence {
              tunnel: w344 -> [w358]
              tunnel: [w355] -> w343
              frame #0 {
                # "Repetition 3"
                n191 = call "Math SubVI - Simple (PCR) (DBG OFF) (SBRTN).vi"("Input"=w358) -> ("Output"=w356:dbl)
                n192 = call "Math SubVI - Medium (PCR) (DBG OFF) (SBRTN).vi"("Input"=w356) -> ("Output"=w357:dbl)
                n193 = call "Math SubVI - Complex (PCR) (DBG OFF) (SBRTN).vi"("Input"=w357) -> ("Output"=w355:dbl)
              }
            }
            n194 = flat-sequence {
              tunnel: w343 -> [w354]
              tunnel: [w351] -> w342
              frame #0 {
                # "Repetition 4"
                n195 = call "Math SubVI - Simple (PCR) (DBG OFF) (SBRTN).vi"("Input"=w354) -> ("Output"=w352:dbl)
                n196 = call "Math SubVI - Medium (PCR) (DBG OFF) (SBRTN).vi"("Input"=w352) -> ("Output"=w353:dbl)
                n197 = call "Math SubVI - Complex (PCR) (DBG OFF) (SBRTN).vi"("Input"=w353) -> ("Output"=w351:dbl)
              }
            }
            n198 = flat-sequence {
              tunnel: w342 -> [w350]
              tunnel: [w347] -> w345
              frame #0 {
                # "Repetition 5"
                n199 = call "Math SubVI - Simple (PCR) (DBG OFF) (SBRTN).vi"("Input"=w350) -> ("Output"=w348:dbl)
                n200 = call "Math SubVI - Medium (PCR) (DBG OFF) (SBRTN).vi"("Input"=w348) -> ("Output"=w349:dbl)
                n201 = call "Math SubVI - Complex (PCR) (DBG OFF) (SBRTN).vi"("Input"=w349) -> ("Output"=w347:dbl)
              }
            }
          }
          frame Enabled {
            # "Case 2: Inline VIs"
            n202 = flat-sequence {
              tunnel: w372 -> [w392]
              tunnel: [w389] -> w371
              frame #0 {
                # "Repetition 1"
                n203 = call "Math SubVI - Simple (PCR) (DBG OFF) (INLN).vi"("Input"=w392) -> ("Output"=w390:dbl)
                n204 = call "Math SubVI - Medium (PCR) (DBG OFF) (INLN).vi"("Input"=w390) -> ("Output"=w391:dbl)
                n205 = call "Math SubVI - Complex (PCR) (DBG OFF) (INLN).vi"("Input"=w391) -> ("Output"=w389:dbl)
              }
            }
            n206 = flat-sequence {
              tunnel: w371 -> [w388]
              tunnel: [w385] -> w370
              frame #0 {
                # "Repetition 2"
                n207 = call "Math SubVI - Simple (PCR) (DBG OFF) (INLN).vi"("Input"=w388) -> ("Output"=w386:dbl)
                n208 = call "Math SubVI - Medium (PCR) (DBG OFF) (INLN).vi"("Input"=w386) -> ("Output"=w387:dbl)
                n209 = call "Math SubVI - Complex (PCR) (DBG OFF) (INLN).vi"("Input"=w387) -> ("Output"=w385:dbl)
              }
            }
            n210 = flat-sequence {
              tunnel: w370 -> [w384]
              tunnel: [w381] -> w369
              frame #0 {
                # "Repetition 3"
                n211 = call "Math SubVI - Simple (PCR) (DBG OFF) (INLN).vi"("Input"=w384) -> ("Output"=w382:dbl)
                n212 = call "Math SubVI - Medium (PCR) (DBG OFF) (INLN).vi"("Input"=w382) -> ("Output"=w383:dbl)
                n213 = call "Math SubVI - Complex (PCR) (DBG OFF) (INLN).vi"("Input"=w383) -> ("Output"=w381:dbl)
              }
            }
            n214 = flat-sequence {
              tunnel: w369 -> [w380]
              tunnel: [w377] -> w368
              frame #0 {
                # "Repetition 4"
                n215 = call "Math SubVI - Simple (PCR) (DBG OFF) (INLN).vi"("Input"=w380) -> ("Output"=w378:dbl)
                n216 = call "Math SubVI - Medium (PCR) (DBG OFF) (INLN).vi"("Input"=w378) -> ("Output"=w379:dbl)
                n217 = call "Math SubVI - Complex (PCR) (DBG OFF) (INLN).vi"("Input"=w379) -> ("Output"=w377:dbl)
              }
            }
            n218 = flat-sequence {
              tunnel: w368 -> [w376]
              tunnel: [w373] -> w367
              frame #0 {
                # "Repetition 5"
                n219 = call "Math SubVI - Simple (PCR) (DBG OFF) (INLN).vi"("Input"=w376) -> ("Output"=w374:dbl)
                n220 = call "Math SubVI - Medium (PCR) (DBG OFF) (INLN).vi"("Input"=w374) -> ("Output"=w375:dbl)
                n221 = call "Math SubVI - Complex (PCR) (DBG OFF) (INLN).vi"("Input"=w375) -> ("Output"=w373:dbl)
              }
            }
          }
        }
        n222 = local read "Stop VI?"() -> (w340:bool)
      }
      n223 = for "Loop 6" {
        N: w22 -> [_]
        tunnel: [w282] -> w32 mode=indexing
        tunnel: [w283] -> w31
        i -> [w283]
        stop <- w284 stop-if-true
        n224 = Random Number (0-1)() -> (number: 0 to 1=w281:dbl)
        n225 = disable-structure shown="Enabled" {
          disable-tunnel: w281 -> [w290 w316]
          disable-tunnel: [w289 w311] -> w282
          frame Disabled {
            # "Case 1: Subroutines"
            n226 = flat-sequence {
              tunnel: w290 -> [w310]
              tunnel: [w307] -> w285
              frame #0 {
                # "Repetition 1"
                n227 = call "Math SubVI - Simple (PCR) (DBG OFF) (SBRTN).vi"("Input"=w310) -> ("Output"=w308:dbl)
                n228 = call "Math SubVI - Medium (PCR) (DBG OFF) (SBRTN).vi"("Input"=w308) -> ("Output"=w309:dbl)
                n229 = call "Math SubVI - Complex (PCR) (DBG OFF) (SBRTN).vi"("Input"=w309) -> ("Output"=w307:dbl)
              }
            }
            n230 = flat-sequence {
              tunnel: w285 -> [w306]
              tunnel: [w303] -> w288
              frame #0 {
                # "Repetition 2"
                n231 = call "Math SubVI - Simple (PCR) (DBG OFF) (SBRTN).vi"("Input"=w306) -> ("Output"=w304:dbl)
                n232 = call "Math SubVI - Medium (PCR) (DBG OFF) (SBRTN).vi"("Input"=w304) -> ("Output"=w305:dbl)
                n233 = call "Math SubVI - Complex (PCR) (DBG OFF) (SBRTN).vi"("Input"=w305) -> ("Output"=w303:dbl)
              }
            }
            n234 = flat-sequence {
              tunnel: w288 -> [w302]
              tunnel: [w299] -> w287
              frame #0 {
                # "Repetition 3"
                n235 = call "Math SubVI - Simple (PCR) (DBG OFF) (SBRTN).vi"("Input"=w302) -> ("Output"=w300:dbl)
                n236 = call "Math SubVI - Medium (PCR) (DBG OFF) (SBRTN).vi"("Input"=w300) -> ("Output"=w301:dbl)
                n237 = call "Math SubVI - Complex (PCR) (DBG OFF) (SBRTN).vi"("Input"=w301) -> ("Output"=w299:dbl)
              }
            }
            n238 = flat-sequence {
              tunnel: w287 -> [w298]
              tunnel: [w295] -> w286
              frame #0 {
                # "Repetition 4"
                n239 = call "Math SubVI - Simple (PCR) (DBG OFF) (SBRTN).vi"("Input"=w298) -> ("Output"=w296:dbl)
                n240 = call "Math SubVI - Medium (PCR) (DBG OFF) (SBRTN).vi"("Input"=w296) -> ("Output"=w297:dbl)
                n241 = call "Math SubVI - Complex (PCR) (DBG OFF) (SBRTN).vi"("Input"=w297) -> ("Output"=w295:dbl)
              }
            }
            n242 = flat-sequence {
              tunnel: w286 -> [w294]
              tunnel: [w291] -> w289
              frame #0 {
                # "Repetition 5"
                n243 = call "Math SubVI - Simple (PCR) (DBG OFF) (SBRTN).vi"("Input"=w294) -> ("Output"=w292:dbl)
                n244 = call "Math SubVI - Medium (PCR) (DBG OFF) (SBRTN).vi"("Input"=w292) -> ("Output"=w293:dbl)
                n245 = call "Math SubVI - Complex (PCR) (DBG OFF) (SBRTN).vi"("Input"=w293) -> ("Output"=w291:dbl)
              }
            }
          }
          frame Enabled {
            # "Case 2: Inline VIs"
            n246 = flat-sequence {
              tunnel: w316 -> [w336]
              tunnel: [w333] -> w315
              frame #0 {
                # "Repetition 1"
                n247 = call "Math SubVI - Simple (PCR) (DBG OFF) (INLN).vi"("Input"=w336) -> ("Output"=w334:dbl)
                n248 = call "Math SubVI - Medium (PCR) (DBG OFF) (INLN).vi"("Input"=w334) -> ("Output"=w335:dbl)
                n249 = call "Math SubVI - Complex (PCR) (DBG OFF) (INLN).vi"("Input"=w335) -> ("Output"=w333:dbl)
              }
            }
            n250 = flat-sequence {
              tunnel: w315 -> [w332]
              tunnel: [w329] -> w314
              frame #0 {
                # "Repetition 2"
                n251 = call "Math SubVI - Simple (PCR) (DBG OFF) (INLN).vi"("Input"=w332) -> ("Output"=w330:dbl)
                n252 = call "Math SubVI - Medium (PCR) (DBG OFF) (INLN).vi"("Input"=w330) -> ("Output"=w331:dbl)
                n253 = call "Math SubVI - Complex (PCR) (DBG OFF) (INLN).vi"("Input"=w331) -> ("Output"=w329:dbl)
              }
            }
            n254 = flat-sequence {
              tunnel: w314 -> [w328]
              tunnel: [w325] -> w313
              frame #0 {
                # "Repetition 3"
                n255 = call "Math SubVI - Simple (PCR) (DBG OFF) (INLN).vi"("Input"=w328) -> ("Output"=w326:dbl)
                n256 = call "Math SubVI - Medium (PCR) (DBG OFF) (INLN).vi"("Input"=w326) -> ("Output"=w327:dbl)
                n257 = call "Math SubVI - Complex (PCR) (DBG OFF) (INLN).vi"("Input"=w327) -> ("Output"=w325:dbl)
              }
            }
            n258 = flat-sequence {
              tunnel: w313 -> [w324]
              tunnel: [w321] -> w312
              frame #0 {
                # "Repetition 4"
                n259 = call "Math SubVI - Simple (PCR) (DBG OFF) (INLN).vi"("Input"=w324) -> ("Output"=w322:dbl)
                n260 = call "Math SubVI - Medium (PCR) (DBG OFF) (INLN).vi"("Input"=w322) -> ("Output"=w323:dbl)
                n261 = call "Math SubVI - Complex (PCR) (DBG OFF) (INLN).vi"("Input"=w323) -> ("Output"=w321:dbl)
              }
            }
            n262 = flat-sequence {
              tunnel: w312 -> [w320]
              tunnel: [w317] -> w311
              frame #0 {
                # "Repetition 5"
                n263 = call "Math SubVI - Simple (PCR) (DBG OFF) (INLN).vi"("Input"=w320) -> ("Output"=w318:dbl)
                n264 = call "Math SubVI - Medium (PCR) (DBG OFF) (INLN).vi"("Input"=w318) -> ("Output"=w319:dbl)
                n265 = call "Math SubVI - Complex (PCR) (DBG OFF) (INLN).vi"("Input"=w319) -> ("Output"=w317:dbl)
              }
            }
          }
        }
        n266 = local read "Stop VI?"() -> (w284:bool)
      }
      n267 = for "Loop 7" {
        N: w22 -> [_]
        tunnel: [w226] -> w30 mode=indexing
        tunnel: [w227] -> w29
        i -> [w227]
        stop <- w228 stop-if-true
        n268 = Random Number (0-1)() -> (number: 0 to 1=w225:dbl)
        n269 = disable-structure shown="Enabled" {
          disable-tunnel: w225 -> [w234 w260]
          disable-tunnel: [w233 w255] -> w226
          frame Disabled {
            # "Case 1: Subroutines"
            n270 = flat-sequence {
              tunnel: w234 -> [w254]
              tunnel: [w251] -> w229
              frame #0 {
                # "Repetition 1"
                n271 = call "Math SubVI - Simple (PCR) (DBG OFF) (SBRTN).vi"("Input"=w254) -> ("Output"=w252:dbl)
                n272 = call "Math SubVI - Medium (PCR) (DBG OFF) (SBRTN).vi"("Input"=w252) -> ("Output"=w253:dbl)
                n273 = call "Math SubVI - Complex (PCR) (DBG OFF) (SBRTN).vi"("Input"=w253) -> ("Output"=w251:dbl)
              }
            }
            n274 = flat-sequence {
              tunnel: w229 -> [w250]
              tunnel: [w247] -> w232
              frame #0 {
                # "Repetition 2"
                n275 = call "Math SubVI - Simple (PCR) (DBG OFF) (SBRTN).vi"("Input"=w250) -> ("Output"=w248:dbl)
                n276 = call "Math SubVI - Medium (PCR) (DBG OFF) (SBRTN).vi"("Input"=w248) -> ("Output"=w249:dbl)
                n277 = call "Math SubVI - Complex (PCR) (DBG OFF) (SBRTN).vi"("Input"=w249) -> ("Output"=w247:dbl)
              }
            }
            n278 = flat-sequence {
              tunnel: w232 -> [w246]
              tunnel: [w243] -> w231
              frame #0 {
                # "Repetition 3"
                n279 = call "Math SubVI - Simple (PCR) (DBG OFF) (SBRTN).vi"("Input"=w246) -> ("Output"=w244:dbl)
                n280 = call "Math SubVI - Medium (PCR) (DBG OFF) (SBRTN).vi"("Input"=w244) -> ("Output"=w245:dbl)
                n281 = call "Math SubVI - Complex (PCR) (DBG OFF) (SBRTN).vi"("Input"=w245) -> ("Output"=w243:dbl)
              }
            }
            n282 = flat-sequence {
              tunnel: w231 -> [w242]
              tunnel: [w239] -> w230
              frame #0 {
                # "Repetition 4"
                n283 = call "Math SubVI - Simple (PCR) (DBG OFF) (SBRTN).vi"("Input"=w242) -> ("Output"=w240:dbl)
                n284 = call "Math SubVI - Medium (PCR) (DBG OFF) (SBRTN).vi"("Input"=w240) -> ("Output"=w241:dbl)
                n285 = call "Math SubVI - Complex (PCR) (DBG OFF) (SBRTN).vi"("Input"=w241) -> ("Output"=w239:dbl)
              }
            }
            n286 = flat-sequence {
              tunnel: w230 -> [w238]
              tunnel: [w235] -> w233
              frame #0 {
                # "Repetition 5"
                n287 = call "Math SubVI - Simple (PCR) (DBG OFF) (SBRTN).vi"("Input"=w238) -> ("Output"=w236:dbl)
                n288 = call "Math SubVI - Medium (PCR) (DBG OFF) (SBRTN).vi"("Input"=w236) -> ("Output"=w237:dbl)
                n289 = call "Math SubVI - Complex (PCR) (DBG OFF) (SBRTN).vi"("Input"=w237) -> ("Output"=w235:dbl)
              }
            }
          }
          frame Enabled {
            # "Case 2: Inline VIs"
            n290 = flat-sequence {
              tunnel: w260 -> [w280]
              tunnel: [w277] -> w259
              frame #0 {
                # "Repetition 1"
                n291 = call "Math SubVI - Simple (PCR) (DBG OFF) (INLN).vi"("Input"=w280) -> ("Output"=w278:dbl)
                n292 = call "Math SubVI - Medium (PCR) (DBG OFF) (INLN).vi"("Input"=w278) -> ("Output"=w279:dbl)
                n293 = call "Math SubVI - Complex (PCR) (DBG OFF) (INLN).vi"("Input"=w279) -> ("Output"=w277:dbl)
              }
            }
            n294 = flat-sequence {
              tunnel: w259 -> [w276]
              tunnel: [w273] -> w258
              frame #0 {
                # "Repetition 2"
                n295 = call "Math SubVI - Simple (PCR) (DBG OFF) (INLN).vi"("Input"=w276) -> ("Output"=w274:dbl)
                n296 = call "Math SubVI - Medium (PCR) (DBG OFF) (INLN).vi"("Input"=w274) -> ("Output"=w275:dbl)
                n297 = call "Math SubVI - Complex (PCR) (DBG OFF) (INLN).vi"("Input"=w275) -> ("Output"=w273:dbl)
              }
            }
            n298 = flat-sequence {
              tunnel: w258 -> [w272]
              tunnel: [w269] -> w257
              frame #0 {
                # "Repetition 3"
                n299 = call "Math SubVI - Simple (PCR) (DBG OFF) (INLN).vi"("Input"=w272) -> ("Output"=w270:dbl)
                n300 = call "Math SubVI - Medium (PCR) (DBG OFF) (INLN).vi"("Input"=w270) -> ("Output"=w271:dbl)
                n301 = call "Math SubVI - Complex (PCR) (DBG OFF) (INLN).vi"("Input"=w271) -> ("Output"=w269:dbl)
              }
            }
            n302 = flat-sequence {
              tunnel: w257 -> [w268]
              tunnel: [w265] -> w256
              frame #0 {
                # "Repetition 4"
                n303 = call "Math SubVI - Simple (PCR) (DBG OFF) (INLN).vi"("Input"=w268) -> ("Output"=w266:dbl)
                n304 = call "Math SubVI - Medium (PCR) (DBG OFF) (INLN).vi"("Input"=w266) -> ("Output"=w267:dbl)
                n305 = call "Math SubVI - Complex (PCR) (DBG OFF) (INLN).vi"("Input"=w267) -> ("Output"=w265:dbl)
              }
            }
            n306 = flat-sequence {
              tunnel: w256 -> [w264]
              tunnel: [w261] -> w255
              frame #0 {
                # "Repetition 5"
                n307 = call "Math SubVI - Simple (PCR) (DBG OFF) (INLN).vi"("Input"=w264) -> ("Output"=w262:dbl)
                n308 = call "Math SubVI - Medium (PCR) (DBG OFF) (INLN).vi"("Input"=w262) -> ("Output"=w263:dbl)
                n309 = call "Math SubVI - Complex (PCR) (DBG OFF) (INLN).vi"("Input"=w263) -> ("Output"=w261:dbl)
              }
            }
          }
        }
        n310 = local read "Stop VI?"() -> (w228:bool)
      }
      n311 = for "Loop 8" {
        N: w22 -> [_]
        tunnel: [w170] -> w27 mode=indexing
        tunnel: [w171] -> w28
        i -> [w171]
        stop <- w172 stop-if-true
        n312 = Random Number (0-1)() -> (number: 0 to 1=w169:dbl)
        n313 = disable-structure shown="Enabled" {
          disable-tunnel: w169 -> [w178 w204]
          disable-tunnel: [w177 w199] -> w170
          frame Disabled {
            # "Case 1: Subroutines"
            n314 = flat-sequence {
              tunnel: w178 -> [w198]
              tunnel: [w195] -> w173
              frame #0 {
                # "Repetition 1"
                n315 = call "Math SubVI - Simple (PCR) (DBG OFF) (SBRTN).vi"("Input"=w198) -> ("Output"=w196:dbl)
                n316 = call "Math SubVI - Medium (PCR) (DBG OFF) (SBRTN).vi"("Input"=w196) -> ("Output"=w197:dbl)
                n317 = call "Math SubVI - Complex (PCR) (DBG OFF) (SBRTN).vi"("Input"=w197) -> ("Output"=w195:dbl)
              }
            }
            n318 = flat-sequence {
              tunnel: w173 -> [w194]
              tunnel: [w191] -> w176
              frame #0 {
                # "Repetition 2"
                n319 = call "Math SubVI - Simple (PCR) (DBG OFF) (SBRTN).vi"("Input"=w194) -> ("Output"=w192:dbl)
                n320 = call "Math SubVI - Medium (PCR) (DBG OFF) (SBRTN).vi"("Input"=w192) -> ("Output"=w193:dbl)
                n321 = call "Math SubVI - Complex (PCR) (DBG OFF) (SBRTN).vi"("Input"=w193) -> ("Output"=w191:dbl)
              }
            }
            n322 = flat-sequence {
              tunnel: w176 -> [w190]
              tunnel: [w187] -> w175
              frame #0 {
                # "Repetition 3"
                n323 = call "Math SubVI - Simple (PCR) (DBG OFF) (SBRTN).vi"("Input"=w190) -> ("Output"=w188:dbl)
                n324 = call "Math SubVI - Medium (PCR) (DBG OFF) (SBRTN).vi"("Input"=w188) -> ("Output"=w189:dbl)
                n325 = call "Math SubVI - Complex (PCR) (DBG OFF) (SBRTN).vi"("Input"=w189) -> ("Output"=w187:dbl)
              }
            }
            n326 = flat-sequence {
              tunnel: w175 -> [w186]
              tunnel: [w183] -> w174
              frame #0 {
                # "Repetition 4"
                n327 = call "Math SubVI - Simple (PCR) (DBG OFF) (SBRTN).vi"("Input"=w186) -> ("Output"=w184:dbl)
                n328 = call "Math SubVI - Medium (PCR) (DBG OFF) (SBRTN).vi"("Input"=w184) -> ("Output"=w185:dbl)
                n329 = call "Math SubVI - Complex (PCR) (DBG OFF) (SBRTN).vi"("Input"=w185) -> ("Output"=w183:dbl)
              }
            }
            n330 = flat-sequence {
              tunnel: w174 -> [w182]
              tunnel: [w179] -> w177
              frame #0 {
                # "Repetition 5"
                n331 = call "Math SubVI - Simple (PCR) (DBG OFF) (SBRTN).vi"("Input"=w182) -> ("Output"=w180:dbl)
                n332 = call "Math SubVI - Medium (PCR) (DBG OFF) (SBRTN).vi"("Input"=w180) -> ("Output"=w181:dbl)
                n333 = call "Math SubVI - Complex (PCR) (DBG OFF) (SBRTN).vi"("Input"=w181) -> ("Output"=w179:dbl)
              }
            }
          }
          frame Enabled {
            # "Case 2: Inline VIs"
            n334 = flat-sequence {
              tunnel: w204 -> [w224]
              tunnel: [w221] -> w203
              frame #0 {
                # "Repetition 1"
                n335 = call "Math SubVI - Simple (PCR) (DBG OFF) (INLN).vi"("Input"=w224) -> ("Output"=w222:dbl)
                n336 = call "Math SubVI - Medium (PCR) (DBG OFF) (INLN).vi"("Input"=w222) -> ("Output"=w223:dbl)
                n337 = call "Math SubVI - Complex (PCR) (DBG OFF) (INLN).vi"("Input"=w223) -> ("Output"=w221:dbl)
              }
            }
            n338 = flat-sequence {
              tunnel: w203 -> [w220]
              tunnel: [w217] -> w202
              frame #0 {
                # "Repetition 2"
                n339 = call "Math SubVI - Simple (PCR) (DBG OFF) (INLN).vi"("Input"=w220) -> ("Output"=w218:dbl)
                n340 = call "Math SubVI - Medium (PCR) (DBG OFF) (INLN).vi"("Input"=w218) -> ("Output"=w219:dbl)
                n341 = call "Math SubVI - Complex (PCR) (DBG OFF) (INLN).vi"("Input"=w219) -> ("Output"=w217:dbl)
              }
            }
            n342 = flat-sequence {
              tunnel: w202 -> [w216]
              tunnel: [w213] -> w201
              frame #0 {
                # "Repetition 3"
                n343 = call "Math SubVI - Simple (PCR) (DBG OFF) (INLN).vi"("Input"=w216) -> ("Output"=w214:dbl)
                n344 = call "Math SubVI - Medium (PCR) (DBG OFF) (INLN).vi"("Input"=w214) -> ("Output"=w215:dbl)
                n345 = call "Math SubVI - Complex (PCR) (DBG OFF) (INLN).vi"("Input"=w215) -> ("Output"=w213:dbl)
              }
            }
            n346 = flat-sequence {
              tunnel: w201 -> [w212]
              tunnel: [w209] -> w200
              frame #0 {
                # "Repetition 4"
                n347 = call "Math SubVI - Simple (PCR) (DBG OFF) (INLN).vi"("Input"=w212) -> ("Output"=w210:dbl)
                n348 = call "Math SubVI - Medium (PCR) (DBG OFF) (INLN).vi"("Input"=w210) -> ("Output"=w211:dbl)
                n349 = call "Math SubVI - Complex (PCR) (DBG OFF) (INLN).vi"("Input"=w211) -> ("Output"=w209:dbl)
              }
            }
            n350 = flat-sequence {
              tunnel: w200 -> [w208]
              tunnel: [w205] -> w199
              frame #0 {
                # "Repetition 5"
                n351 = call "Math SubVI - Simple (PCR) (DBG OFF) (INLN).vi"("Input"=w208) -> ("Output"=w206:dbl)
                n352 = call "Math SubVI - Medium (PCR) (DBG OFF) (INLN).vi"("Input"=w206) -> ("Output"=w207:dbl)
                n353 = call "Math SubVI - Complex (PCR) (DBG OFF) (INLN).vi"("Input"=w207) -> ("Output"=w205:dbl)
              }
            }
          }
        }
        n354 = local read "Stop VI?"() -> (w172:bool)
      }
      n355 = for "Loop 9" {
        N: w22 -> [_]
        tunnel: [w114] -> w25 mode=indexing
        tunnel: [w115] -> w26
        i -> [w115]
        stop <- w116 stop-if-true
        n356 = Random Number (0-1)() -> (number: 0 to 1=w113:dbl)
        n357 = disable-structure shown="Enabled" {
          disable-tunnel: w113 -> [w122 w148]
          disable-tunnel: [w121 w143] -> w114
          frame Disabled {
            # "Case 1: Subroutines"
            n358 = flat-sequence {
              tunnel: w122 -> [w142]
              tunnel: [w139] -> w117
              frame #0 {
                # "Repetition 1"
                n359 = call "Math SubVI - Simple (PCR) (DBG OFF) (SBRTN).vi"("Input"=w142) -> ("Output"=w140:dbl)
                n360 = call "Math SubVI - Medium (PCR) (DBG OFF) (SBRTN).vi"("Input"=w140) -> ("Output"=w141:dbl)
                n361 = call "Math SubVI - Complex (PCR) (DBG OFF) (SBRTN).vi"("Input"=w141) -> ("Output"=w139:dbl)
              }
            }
            n362 = flat-sequence {
              tunnel: w117 -> [w138]
              tunnel: [w135] -> w120
              frame #0 {
                # "Repetition 2"
                n363 = call "Math SubVI - Simple (PCR) (DBG OFF) (SBRTN).vi"("Input"=w138) -> ("Output"=w136:dbl)
                n364 = call "Math SubVI - Medium (PCR) (DBG OFF) (SBRTN).vi"("Input"=w136) -> ("Output"=w137:dbl)
                n365 = call "Math SubVI - Complex (PCR) (DBG OFF) (SBRTN).vi"("Input"=w137) -> ("Output"=w135:dbl)
              }
            }
            n366 = flat-sequence {
              tunnel: w120 -> [w134]
              tunnel: [w131] -> w119
              frame #0 {
                # "Repetition 3"
                n367 = call "Math SubVI - Simple (PCR) (DBG OFF) (SBRTN).vi"("Input"=w134) -> ("Output"=w132:dbl)
                n368 = call "Math SubVI - Medium (PCR) (DBG OFF) (SBRTN).vi"("Input"=w132) -> ("Output"=w133:dbl)
                n369 = call "Math SubVI - Complex (PCR) (DBG OFF) (SBRTN).vi"("Input"=w133) -> ("Output"=w131:dbl)
              }
            }
            n370 = flat-sequence {
              tunnel: w119 -> [w130]
              tunnel: [w127] -> w118
              frame #0 {
                # "Repetition 4"
                n371 = call "Math SubVI - Simple (PCR) (DBG OFF) (SBRTN).vi"("Input"=w130) -> ("Output"=w128:dbl)
                n372 = call "Math SubVI - Medium (PCR) (DBG OFF) (SBRTN).vi"("Input"=w128) -> ("Output"=w129:dbl)
                n373 = call "Math SubVI - Complex (PCR) (DBG OFF) (SBRTN).vi"("Input"=w129) -> ("Output"=w127:dbl)
              }
            }
            n374 = flat-sequence {
              tunnel: w118 -> [w126]
              tunnel: [w123] -> w121
              frame #0 {
                # "Repetition 5"
                n375 = call "Math SubVI - Simple (PCR) (DBG OFF) (SBRTN).vi"("Input"=w126) -> ("Output"=w124:dbl)
                n376 = call "Math SubVI - Medium (PCR) (DBG OFF) (SBRTN).vi"("Input"=w124) -> ("Output"=w125:dbl)
                n377 = call "Math SubVI - Complex (PCR) (DBG OFF) (SBRTN).vi"("Input"=w125) -> ("Output"=w123:dbl)
              }
            }
          }
          frame Enabled {
            # "Case 2: Inline VIs"
            n378 = flat-sequence {
              tunnel: w148 -> [w168]
              tunnel: [w165] -> w147
              frame #0 {
                # "Repetition 1"
                n379 = call "Math SubVI - Simple (PCR) (DBG OFF) (INLN).vi"("Input"=w168) -> ("Output"=w166:dbl)
                n380 = call "Math SubVI - Medium (PCR) (DBG OFF) (INLN).vi"("Input"=w166) -> ("Output"=w167:dbl)
                n381 = call "Math SubVI - Complex (PCR) (DBG OFF) (INLN).vi"("Input"=w167) -> ("Output"=w165:dbl)
              }
            }
            n382 = flat-sequence {
              tunnel: w147 -> [w164]
              tunnel: [w161] -> w146
              frame #0 {
                # "Repetition 2"
                n383 = call "Math SubVI - Simple (PCR) (DBG OFF) (INLN).vi"("Input"=w164) -> ("Output"=w162:dbl)
                n384 = call "Math SubVI - Medium (PCR) (DBG OFF) (INLN).vi"("Input"=w162) -> ("Output"=w163:dbl)
                n385 = call "Math SubVI - Complex (PCR) (DBG OFF) (INLN).vi"("Input"=w163) -> ("Output"=w161:dbl)
              }
            }
            n386 = flat-sequence {
              tunnel: w146 -> [w160]
              tunnel: [w157] -> w145
              frame #0 {
                # "Repetition 3"
                n387 = call "Math SubVI - Simple (PCR) (DBG OFF) (INLN).vi"("Input"=w160) -> ("Output"=w158:dbl)
                n388 = call "Math SubVI - Medium (PCR) (DBG OFF) (INLN).vi"("Input"=w158) -> ("Output"=w159:dbl)
                n389 = call "Math SubVI - Complex (PCR) (DBG OFF) (INLN).vi"("Input"=w159) -> ("Output"=w157:dbl)
              }
            }
            n390 = flat-sequence {
              tunnel: w145 -> [w156]
              tunnel: [w153] -> w144
              frame #0 {
                # "Repetition 4"
                n391 = call "Math SubVI - Simple (PCR) (DBG OFF) (INLN).vi"("Input"=w156) -> ("Output"=w154:dbl)
                n392 = call "Math SubVI - Medium (PCR) (DBG OFF) (INLN).vi"("Input"=w154) -> ("Output"=w155:dbl)
                n393 = call "Math SubVI - Complex (PCR) (DBG OFF) (INLN).vi"("Input"=w155) -> ("Output"=w153:dbl)
              }
            }
            n394 = flat-sequence {
              tunnel: w144 -> [w152]
              tunnel: [w149] -> w143
              frame #0 {
                # "Repetition 5"
                n395 = call "Math SubVI - Simple (PCR) (DBG OFF) (INLN).vi"("Input"=w152) -> ("Output"=w150:dbl)
                n396 = call "Math SubVI - Medium (PCR) (DBG OFF) (INLN).vi"("Input"=w150) -> ("Output"=w151:dbl)
                n397 = call "Math SubVI - Complex (PCR) (DBG OFF) (INLN).vi"("Input"=w151) -> ("Output"=w149:dbl)
              }
            }
          }
        }
        n398 = local read "Stop VI?"() -> (w116:bool)
      }
      n399 = for "Loop 10" {
        N: w22 -> [_]
        tunnel: [w58] -> w23 mode=indexing
        tunnel: [w59] -> w24
        i -> [w59]
        stop <- w60 stop-if-true
        n400 = Random Number (0-1)() -> (number: 0 to 1=w57:dbl)
        n401 = disable-structure shown="Enabled" {
          disable-tunnel: w57 -> [w66 w92]
          disable-tunnel: [w65 w87] -> w58
          frame Disabled {
            # "Case 1: Subroutines"
            n402 = flat-sequence {
              tunnel: w66 -> [w86]
              tunnel: [w83] -> w61
              frame #0 {
                # "Repetition 1"
                n403 = call "Math SubVI - Simple (PCR) (DBG OFF) (SBRTN).vi"("Input"=w86) -> ("Output"=w84:dbl)
                n404 = call "Math SubVI - Medium (PCR) (DBG OFF) (SBRTN).vi"("Input"=w84) -> ("Output"=w85:dbl)
                n405 = call "Math SubVI - Complex (PCR) (DBG OFF) (SBRTN).vi"("Input"=w85) -> ("Output"=w83:dbl)
              }
            }
            n406 = flat-sequence {
              tunnel: w61 -> [w82]
              tunnel: [w79] -> w64
              frame #0 {
                # "Repetition 2"
                n407 = call "Math SubVI - Simple (PCR) (DBG OFF) (SBRTN).vi"("Input"=w82) -> ("Output"=w80:dbl)
                n408 = call "Math SubVI - Medium (PCR) (DBG OFF) (SBRTN).vi"("Input"=w80) -> ("Output"=w81:dbl)
                n409 = call "Math SubVI - Complex (PCR) (DBG OFF) (SBRTN).vi"("Input"=w81) -> ("Output"=w79:dbl)
              }
            }
            n410 = flat-sequence {
              tunnel: w64 -> [w78]
              tunnel: [w75] -> w63
              frame #0 {
                # "Repetition 3"
                n411 = call "Math SubVI - Simple (PCR) (DBG OFF) (SBRTN).vi"("Input"=w78) -> ("Output"=w76:dbl)
                n412 = call "Math SubVI - Medium (PCR) (DBG OFF) (SBRTN).vi"("Input"=w76) -> ("Output"=w77:dbl)
                n413 = call "Math SubVI - Complex (PCR) (DBG OFF) (SBRTN).vi"("Input"=w77) -> ("Output"=w75:dbl)
              }
            }
            n414 = flat-sequence {
              tunnel: w63 -> [w74]
              tunnel: [w71] -> w62
              frame #0 {
                # "Repetition 4"
                n415 = call "Math SubVI - Simple (PCR) (DBG OFF) (SBRTN).vi"("Input"=w74) -> ("Output"=w72:dbl)
                n416 = call "Math SubVI - Medium (PCR) (DBG OFF) (SBRTN).vi"("Input"=w72) -> ("Output"=w73:dbl)
                n417 = call "Math SubVI - Complex (PCR) (DBG OFF) (SBRTN).vi"("Input"=w73) -> ("Output"=w71:dbl)
              }
            }
            n418 = flat-sequence {
              tunnel: w62 -> [w70]
              tunnel: [w67] -> w65
              frame #0 {
                # "Repetition 5"
                n419 = call "Math SubVI - Simple (PCR) (DBG OFF) (SBRTN).vi"("Input"=w70) -> ("Output"=w68:dbl)
                n420 = call "Math SubVI - Medium (PCR) (DBG OFF) (SBRTN).vi"("Input"=w68) -> ("Output"=w69:dbl)
                n421 = call "Math SubVI - Complex (PCR) (DBG OFF) (SBRTN).vi"("Input"=w69) -> ("Output"=w67:dbl)
              }
            }
          }
          frame Enabled {
            # "Case 2: Inline VIs"
            n422 = flat-sequence {
              tunnel: w92 -> [w112]
              tunnel: [w109] -> w91
              frame #0 {
                # "Repetition 1"
                n423 = call "Math SubVI - Simple (PCR) (DBG OFF) (INLN).vi"("Input"=w112) -> ("Output"=w110:dbl)
                n424 = call "Math SubVI - Medium (PCR) (DBG OFF) (INLN).vi"("Input"=w110) -> ("Output"=w111:dbl)
                n425 = call "Math SubVI - Complex (PCR) (DBG OFF) (INLN).vi"("Input"=w111) -> ("Output"=w109:dbl)
              }
            }
            n426 = flat-sequence {
              tunnel: w91 -> [w108]
              tunnel: [w105] -> w90
              frame #0 {
                # "Repetition 2"
                n427 = call "Math SubVI - Simple (PCR) (DBG OFF) (INLN).vi"("Input"=w108) -> ("Output"=w106:dbl)
                n428 = call "Math SubVI - Medium (PCR) (DBG OFF) (INLN).vi"("Input"=w106) -> ("Output"=w107:dbl)
                n429 = call "Math SubVI - Complex (PCR) (DBG OFF) (INLN).vi"("Input"=w107) -> ("Output"=w105:dbl)
              }
            }
            n430 = flat-sequence {
              tunnel: w90 -> [w104]
              tunnel: [w101] -> w89
              frame #0 {
                # "Repetition 3"
                n431 = call "Math SubVI - Simple (PCR) (DBG OFF) (INLN).vi"("Input"=w104) -> ("Output"=w102:dbl)
                n432 = call "Math SubVI - Medium (PCR) (DBG OFF) (INLN).vi"("Input"=w102) -> ("Output"=w103:dbl)
                n433 = call "Math SubVI - Complex (PCR) (DBG OFF) (INLN).vi"("Input"=w103) -> ("Output"=w101:dbl)
              }
            }
            n434 = flat-sequence {
              tunnel: w89 -> [w100]
              tunnel: [w97] -> w88
              frame #0 {
                # "Repetition 4"
                n435 = call "Math SubVI - Simple (PCR) (DBG OFF) (INLN).vi"("Input"=w100) -> ("Output"=w98:dbl)
                n436 = call "Math SubVI - Medium (PCR) (DBG OFF) (INLN).vi"("Input"=w98) -> ("Output"=w99:dbl)
                n437 = call "Math SubVI - Complex (PCR) (DBG OFF) (INLN).vi"("Input"=w99) -> ("Output"=w97:dbl)
              }
            }
            n438 = flat-sequence {
              tunnel: w88 -> [w96]
              tunnel: [w93] -> w87
              frame #0 {
                # "Repetition 5"
                n439 = call "Math SubVI - Simple (PCR) (DBG OFF) (INLN).vi"("Input"=w96) -> ("Output"=w94:dbl)
                n440 = call "Math SubVI - Medium (PCR) (DBG OFF) (INLN).vi"("Input"=w94) -> ("Output"=w95:dbl)
                n441 = call "Math SubVI - Complex (PCR) (DBG OFF) (INLN).vi"("Input"=w95) -> ("Output"=w93:dbl)
              }
            }
          }
        }
        n442 = local read "Stop VI?"() -> (w60:bool)
      }
      n443 = call <vilib>:"High Resolution Polling Wait.vi"("seconds to wait"=w54) -> ("error out"=w53:errorcluster)  [unwired: 10 in]
      n444 = flat-sequence {
        tunnel: w53 -> [w55]
        frame #0 {
          n445 = call <vilib>:"Clear Errors.vi"("error in (no error)"=w55) -> ()  [unwired: 5 in, 2 out]
          "Stop VI?" <- TRUE
        }
      }
      n446 = Increment(x=w33) -> (x+1=w46:i32)
      n447 = Increment(x=w31) -> (x+1=w41:i32)
      n448 = Increment(x=w29) -> (x+1=w42:i32)
      n449 = Increment(x=w28) -> (x+1=w43:i32)
      n450 = Increment(x=w26) -> (x+1=w44:i32)
      n451 = Increment(x=w24) -> (x+1=w45:i32)
      n452 = Increment(x=w51) -> (x+1=w50:i32)
      n453 = Increment(x=w39) -> (x+1=w49:i32)
      n454 = Increment(x=w37) -> (x+1=w48:i32)
      n455 = Increment(x=w35) -> (x+1=w47:i32)
    }
    frame #2 {
      n456 = Build Array(w641, w640, w636, w635, w627, w626, w625, w624, w623, w622) -> (w621:i32[])
      n457 = for {
        tunnel: w621 -> [w647] mode=indexing
        tunnel: [w646] -> w620 mode=indexing
        n458 = Number To Decimal String(number=w647) -> (decimal integer string=w646:string)  [unwired: 1 in]
      }
      n459 = To Double Precision Float(number=w621) -> (double precision float=w634:dbl[])
      n460 = call-poly <vilib>:"Mean.vi"("X"=w634) -> ("mean"=w639:dbl)  [unwired: 1 out]
      "Avg. No. Of Iterations Executed - All Loops" <- w639
      n461 = disable-structure shown="Enabled" {
        disable-tunnel: w639 -> [w645 _]
        frame Disabled {
          n462 = call "Copy Result To Clipboard.vi"("No. Of Decimal Places (6)"=u32 1, "Input"=w645) -> ()
        }
        frame Enabled {
        }
      }
      n463 = call-poly <vilib>:"1D String Array to Delimited String.vi"("delimiter"="\r\n", "string array"=w620) -> ("delimited string"=w617:string)  [unwired: 9 in]
      "No. Of Iterations As Block Of Text (easy to copy into Excel)" <- w617
      n464 = invoke class="Application" method="Clipboard.Write"("Param 0"=w617) -> (error out=w618:errorcluster)  [unwired: 3 in, 3 out]
      n465 = call <vilib>:"Clear Errors.vi"("error in (no error)"=w618) -> ()  [unwired: 5 in, 2 out]
      "No. Of Iterations Executed - Loop 1" <- w641
      "Output - Loop 1" <- w643
      "No. Of Iterations Executed - Loop 2" <- w640
      "Output - Loop 2" <- w642
      "No. Of Iterations Executed - Loop 3" <- w636
      "Output - Loop 3" <- w638
      "No. Of Iterations Executed - Loop 4" <- w635
      "Output - Loop 4" <- w637
      "No. Of Iterations Executed - Loop 5" <- w627
      "Output - Loop 5" <- w633
      "No. Of Iterations Executed - Loop 6" <- w626
      "Output - Loop 6" <- w632
      "No. Of Iterations Executed - Loop 7" <- w625
      "Output - Loop 7" <- w631
      "No. Of Iterations Executed - Loop 8" <- w624
      "Output - Loop 8" <- w630
      "No. Of Iterations Executed - Loop 9" <- w623
      "Output - Loop 9" <- w629
      "No. Of Iterations Executed - Loop 10" <- w622
      "Output - Loop 10" <- w628
    }
  }
